vi "AMC Dispatch Get All Queues.vi"(8 "error in (no error)":errorcluster, 11 "receiver host":string) -> (0 "error out":errorcluster, 2 "String Response":string)   [LabVIEW 2017]
uses:
  subVIs/amc_Globals.vi
  Tools/Keyed Array/Tools_KeyedArray KeyedArray.ctl
  subVIs/TypeDefs/amc_Message.ctl
panel:
  out "Message":T1
  in  "Timeout (100 ms)":i32=1000
  out "Response time (ms)":i32
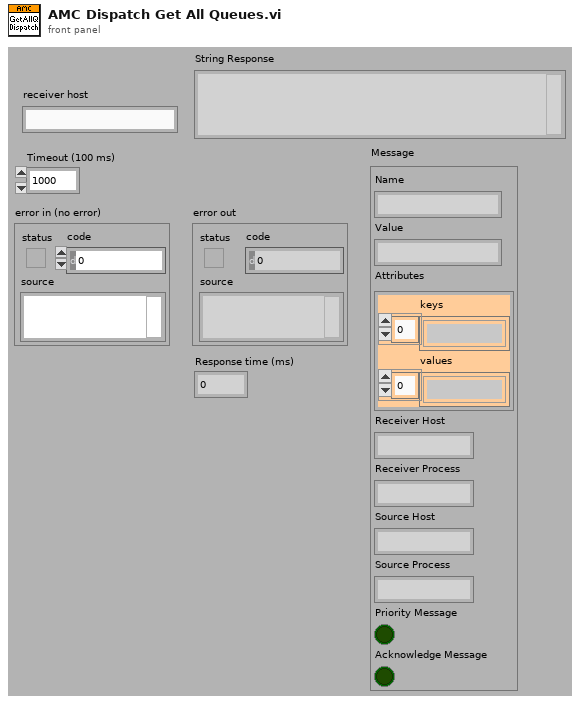
[diagram p1: front panel]
types:
  T1 = typedef "amc_Message.ctl" = cluster{"Name":string, "Value":string, "Attributes":T2, "Receiver Host":string, "Receiver Process":string, "Source Host":string, "Source Process":string, "Priority Message":bool, "Acknowledge Message":bool}
  T2 = typedef "Tools_KeyedArray KeyedArray.ctl" = cluster{"keys":string[], "values":string[]}
  T3 = typedef "amc_Message Queue.ctl" = refnum<queue>
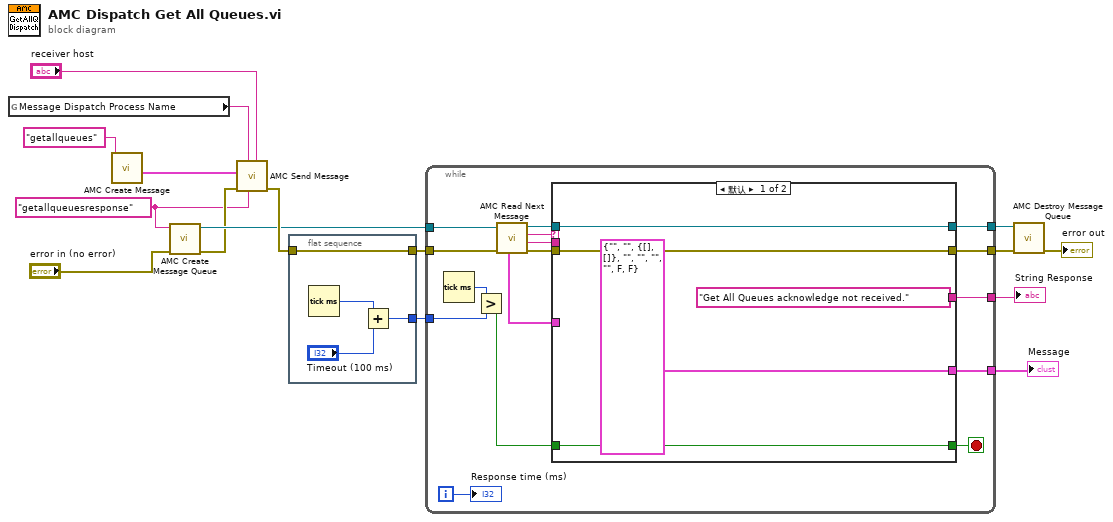
[diagram p0: block diagram]
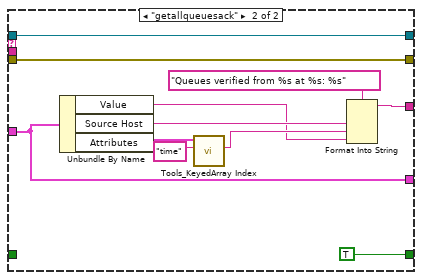
[diagram p2: hidden frame]
diagram:
  w3 = "getallqueuesresponse" ("message queue name")
  n1 = global read "amc_Globals.vi" "Message Dispatch Process Name"() -> (w1:string)
  n2 = call "AMC Create Message.vi"("Name"="getallqueues") -> ("Message"=w5:T1)  [unwired: 2 in, 8 out]
  n3 = call "AMC Create Message Queue.vi"("error in (no error)"="error in (no error)", "Message Queue Name"=w3) -> ("error out"=w6:errorcluster, "Message Queue out"=w7:T3)  [unwired: 2 in, 6 out]
  n4 = call "AMC Send Message.vi"("Receiver Host"="receiver host", "Source Process"=w3, "Receiver Process"=w1, "error in (no error)"=w6, "Message"=w5) -> ("error out"=w12:errorcluster)  [unwired: 3 in, 3 out]
  n5 = flat-sequence {
    tunnel: [w20] -> w11
    tunnel: w12 -> [w20]
    tunnel: [w17] -> w10
    frame #0 {
      n6 = Tick Count (ms)() -> (millisecond timer value=w19:u32)
      n7 = Add(x=w19, y="Timeout (100 ms)") -> (x+y=w17:u32)
    }
  }
  n8 = while {
    tunnel: w11 -> [w36]
    tunnel: [w33] -> w14
    tunnel: [w32] -> w4
    tunnel: [w29] -> w8
    tunnel: [w28] -> w9
    tunnel: w7 -> [w27]
    tunnel: w10 -> [w25]
    i -> [w22]
    stop <- w24 stop-if-true
    n9 = Tick Count (ms)() -> (millisecond timer value=w26:u32)
    n10 = Greater?(x=w26, y=w25) -> (0:w23:bool)
    n11 = call "AMC Read Next Message.vi"("error in (no error)"=w36, "Message Queue in"=w27) -> ("error out"=w31:errorcluster, "Message Value"=w21:string, "Message Name"=w35:string, "Message Queue out"=w30:T3, "Message"=w34:T1)  [unwired: 2 in, 3 out]
    n12 = case shown="默认" w35 {
      tunnel: w34 -> [_ w51]
      tunnel: ["Get All Queues acknowledge not received." w52] -> w33
      tunnel: [T1 {"Name"="", "Value"="", "Attributes"={"keys"=[], "values"=[]}, "Receiver Host"="", "Receiver Process"="", "Source Host"="", "Source Process"="", "Priority Message"=FALSE, "Acknowledge Message"=FALSE} ("Message") w51] -> w32
      tunnel: [w38 w50] -> w29
      tunnel: w31 -> [w38 w50]
      tunnel: [w39 w49] -> w28
      tunnel: w30 -> [w39 w49]
      tunnel: [w37 TRUE] -> w24
      tunnel: w23 -> [w37 _]
      tunnel: w21 -> [_ _]
      frame Default {
      }
      frame "getallqueuesack" {
        n13 = Unbundle By Name(w51) -> ("Value"=w42:string, "Source Host"=w44:string, "Attributes"=w45:T2)
        n14 = call "Tools_KeyedArray Index.vi"("key"="time", "array in"=w45) -> ("value"=w43:string)  [unwired: 2 in, 3 out]
        n15 = Format Into String(format string="Queues verified from %s at %s: %s", w44, w43, w42) -> (resulting string=w52:string)  [unwired: 2 in, 1 out]
      }
    }
    "Response time (ms)" <- w22
  }
  "String Response" <- w14
  "Message" <- w4
  n16 = call "AMC Destroy Message Queue.vi"("error in (no error)"=w8, "Message Queue in"=w9) -> ("error out"=→"error out":errorcluster)  [unwired: 9 out]
